vi "Get Async Loop Rate.vi"(8 "error in (no error)":errorcluster, 11 "Execution Unit in":refnum<class "Execution Unit.lvclass">) -> (0 "error out":errorcluster, 2 "Loop Rate Hz":dbl, 3 "Execution Unit out":refnum<class "Execution Unit.lvclass">)   [LabVIEW 2020, in "AIM ARINC 664 Engine.lvlib" / "Implementation.lvlib" / "Execution Unit.lvclass"]
uses:
  Execution Unit.lvclass
  Execution Unit.lvclass/Execution Unit.ctl
  <vilib>/Utility/SystemLogging/NI_SystemLogging.lvlib
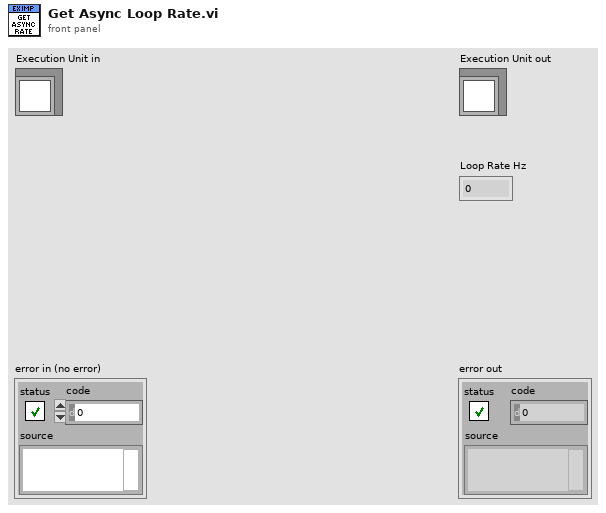
[diagram p1: front panel]
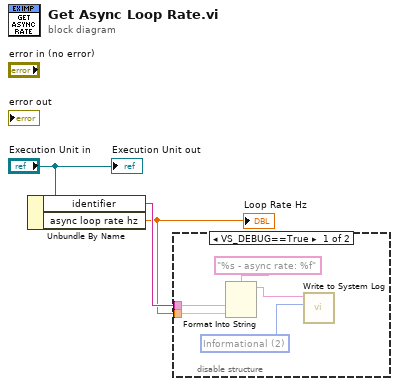
[diagram p0: block diagram]
diagram:
  n1 = Unbundle By Name("Execution Unit in") -> ("identifier"=w2:string, "async loop rate hz"=w1:dbl)
  "Loop Rate Hz" <- w1
  n2 = disable-structure shown="VS_DEBUG==True" {
    disable-tunnel: w2 -> [w8 _]
    disable-tunnel: w1 -> [w7 _]
    frame condition #0 {
      w4 = 2 items=["Error", "Warning", "Informational"] ("severity")
      n3 = Format Into String(format string="%s - async rate: %f", w8, w7) -> (resulting string=w5:string)  [unwired: 2 in, 1 out]
      n4 = call <vilib>:"Write to System Log.vi"("severity"=w4, "message"=w5) -> ()  [unwired: 9 in, 1 out]
    }
    frame condition #1 (active) {
    }
  }
  "Execution Unit out" <- "Execution Unit in"
